vi "Send Launch Functions Message.vi"(6 "Show FP?":bool, 7 "Master?":bool, 8 "error in (no error)":errorcluster, 9 "Device Names":refnum<class "DevInfo.lvclass">[](array[class]), 10 "Function Name":string, 11 "Self Enqueuer In":refnum<class "Message Enqueuer.lvclass">) -> (0 "error out":errorcluster, 3 "Self Enqueuer Out":refnum<class "Message Enqueuer.lvclass">)   [LabVIEW 2016, in "Controller Actor.lvlib" / "Launch Functions Message.lvclass"]
uses:
  <userlib>/Common Components/Controller/Messages/Launch Functions Message/Launch Functions Message.lvclass
  <userlib>/Common Components/Hardware/DevInfo/DevInfo.lvclass
  <vilib>/ActorFramework/Message Enqueuer/Message Enqueuer.lvclass
  C:/Program Files (x86)/National Instruments/LabVIEW 2016/vi.lib/ActorFramework/Message/Message.lvclass
  <userlib>/Common Components/Controller/Messages/Launch Functions Message/Launch Functions Message.lvclass/Launch Functions Message.ctl
  <vilib>/ActorFramework/Message Enqueuer/Message Enqueuer.lvclass/Message Enqueuer.ctl
  <vilib>/ActorFramework/Message Priority Queue/Priority Enqueue.vi
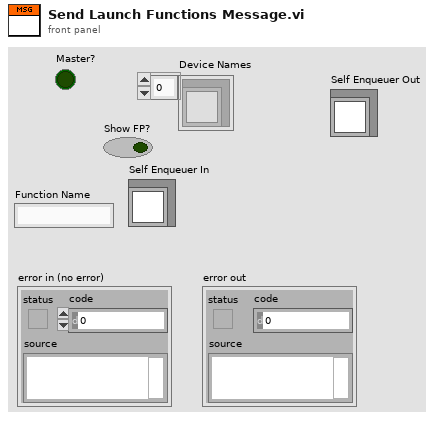
[diagram p1: front panel]
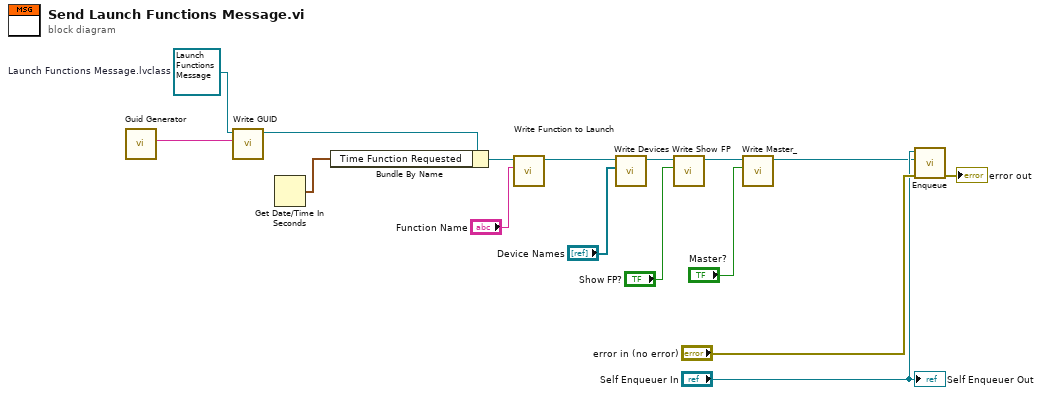
[diagram p0: block diagram]
diagram:
  w7 = refnum<class "Launch Functions Message.lvclass"> refnum  # Launch Functions Message.lvclass
  n1 = call <vilib>:"Guid Generator.vi"() -> ("GUID"=w3:string)  [unwired: 10 in, 1 out]
  n2 = call <userlib>:"Write GUID.vi"("GUID"=w3, "Launch Functions Message in"=w7) -> ("Launch Functions Message out"=w4:refnum<class "Launch Functions Message.lvclass">)  [unwired: 8 in, 1 out]
  n3 = Get Date/Time In Seconds() -> (seconds since 1Jan1904=w5:timestamp)
  n4 = Bundle By Name(cluster=w4, "Time Function Requested"=w5) -> (w6:refnum<class "Launch Functions Message.lvclass">)
  n5 = call <userlib>:"Write Function to Launch.vi"("Function Name"="Function Name", "Launch Functions Message in"=w6) -> ("Launch Functions Message out"=w15:refnum<class "Launch Functions Message.lvclass">)  [unwired: 8 in, 1 out]
  n6 = call <userlib>:"Write Devices.vi"("Devices"="Device Names", "Launch Functions Message in"=w15) -> ("Launch Functions Message out"=w12:refnum<class "Launch Functions Message.lvclass">)  [unwired: 8 in, 1 out]
  n7 = call <userlib>:"Write Show FP.vi"("Show FP?"="Show FP?", "Launch Functions Message in"=w12) -> ("Launch Functions Message out"=w11:refnum<class "Launch Functions Message.lvclass">)  [unwired: 8 in, 1 out]
  n8 = call <userlib>:"Write Master_.vi"("Master?"="Master?", "Launch Functions Message in"=w11) -> ("Launch Functions Message out"=w2:refnum<class "Launch Functions Message.lvclass">)  [unwired: 8 in, 1 out]
  n9 = call <vilib>:"Enqueue.vi"("error in (no error)"="error in (no error)", "Message"=w2, "Message Enqueuer in"="Self Enqueuer In") -> ("error out"=→"error out":errorcluster)  [unwired: 7 in, 1 out]
  "Self Enqueuer Out" <- "Self Enqueuer In"
